vi "LEIN CMD read STATs by len.vi"(0 "SID":u8, 1 "LEIN Variation":T3, 5 "Expected LEN":u16, 7 "STAT ID":u8, 11 "error in":errorcluster) -> (8 "STATs":T1[](array[typedef]), 15 "error out":errorcluster)   [LabVIEW 2011]
uses:
  Defenitions/LEIN Structure variations.ctl
  Defenitions/LEIN CMD Cluster.ctl
  Defenitions/LEIN CMD List.ctl
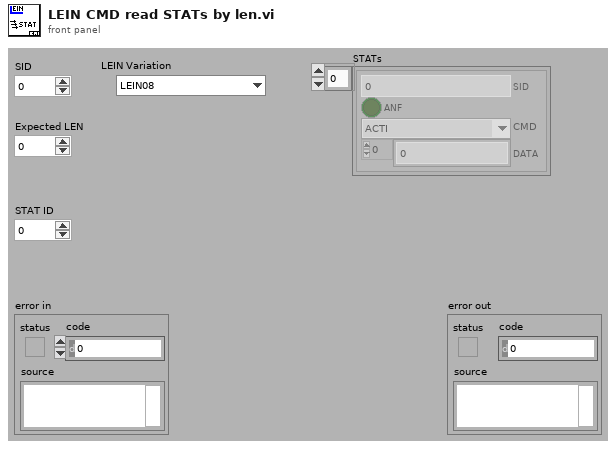
[diagram p1: front panel]
types:
  T1 = typedef "LEIN CMD Cluster.ctl" = cluster{"SID":u8, "ANF":bool, "CMD":T2, "DATA":u8[]}
  T2 = typedef "LEIN CMD List.ctl" = enum8{"ACTI", "TASK", "RES0", "STAT", "RES1", "RES2", "RES3", "USER"}
  T3 = typedef "LEIN Structure variations.ctl" = enum16{"LEIN08", "LEIN31", "LEIN63"}
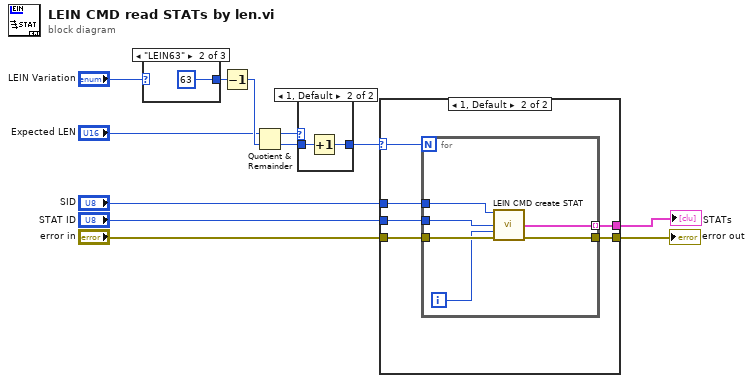
[diagram p0: block diagram]
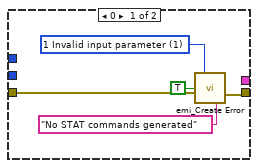
[diagram p2: hidden frame]
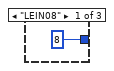
[diagram p4: hidden frame]
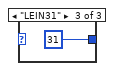
[diagram p5: hidden frame]
diagram:
  n1 = case shown="\"LEIN63\"" "LEIN Variation" {
    tunnel: [8 ("y") 63 ("y") 31 ("y")] -> w7
    frame "LEIN08" {
    }
    frame "LEIN63" {
    }
    frame "LEIN31" {
    }
  }
  n2 = Decrement(x=w7) -> (x-1=w6:i32)
  n3 = Quotient & Remainder(x="Expected LEN", y=w6) -> (x-y*floor(x/y)=w4:i32, floor(x/y)=w3:i32)
  n4 = case shown="1, Default" w4 {
    tunnel: w3 -> [w16 w18]
    tunnel: [w16 w17] -> w2
    frame 0 {
    }
    frame 1, Default {
      n5 = Increment(x=w18) -> (x+1=w17:i32)
    }
  }
  n6 = case shown="1, Default" w2 {
    selector: w2 -> [_ w25]
    tunnel: [w20 w29] -> w12
    tunnel: "STAT ID" -> [_ w28]
    tunnel: "SID" -> [_ w27]
    tunnel: "error in" -> [w21 w26]
    tunnel: [_ w24] -> w1
    frame 0 {
      w23 = 1 items=["0 No Error"=0, "1 Invalid input parameter"=1, "6 Generic file IO "=6, "7 File not Found"=7, "35 Generic Pring Error"=35, "37 Device not Found"=37, "39 Device Unit Error"=39, "40 Could fot Open Device"=40, "42 Generic Error"=42, "52 Unknown Message"=52, "98 Bad File type"=98, "99 Bad File Version"=99, "100 Bad Data in File"=100, "1018 Unspecefied Error"=1018, "1041 Incorrect Password"=1041, "1043 Feature not in this version"=1043, "1109 Unsuported Data type"=1109, "1444 Did not close sucessfully"=1444] ("Error Code")
      n7 = call "emi_Create Error.vi"("Error Code"=w23, "Error(T)"=TRUE, "error in (no error)"=w21, "Append String(\"\")"="No STAT commands generated" ("Append String(\"\")")) -> ("error out"=w20:errorcluster)  [unwired: 11 in]
    }
    frame 1, Default {
      n8 = for {
        N: w25 -> [_]
        tunnel: [w35] -> w29
        tunnel: w28 -> [w34]
        tunnel: w27 -> [w33]
        tunnel: w26 -> [w32]
        tunnel: [w31] -> w24 mode=indexing
        i -> [w30]
        n9 = call "LEIN CMD create STAT.vi"("SID"=w33, "STAT ID"=w34, "STAT Part"=w30, "error in (no error)"=w32) -> ("CMD"=w31:T1, "error out"=w35:errorcluster)  [unwired: 10 in]
      }
    }
  }
  "error out" <- w12
  "STATs" <- w1
